vi "CNR find scaling parameters.vi"(10 "parameters":dbl[](array[numeric]), 11 "old parameter scale factors":dbl[](array[numeric])) -> (3 "parameter scale factors":dbl[](array[numeric]))   [LabVIEW 2017, in "NI_Gmath.lvlib"]
uses:
  <vilib>/gmath/NI_Gmath.lvlib
panel:
  in  "scale params?":bool=TRUE
  out "x*y":dbl[](array[numeric])
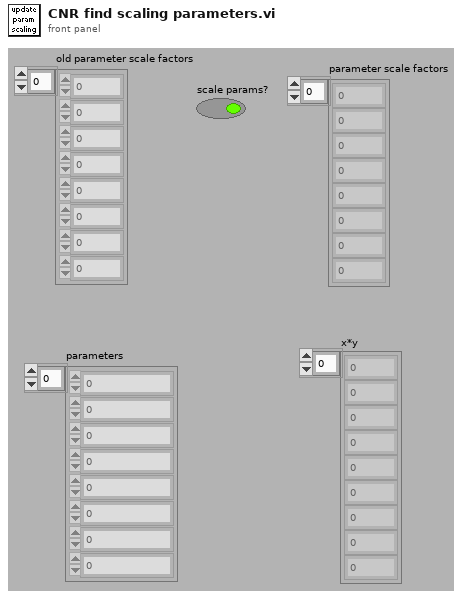
[diagram p1: front panel]
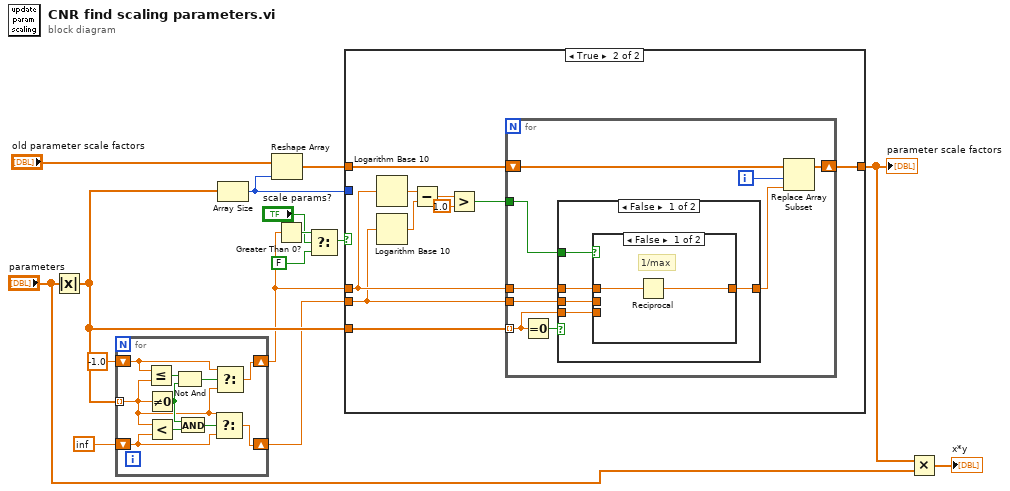
[diagram p0: block diagram]
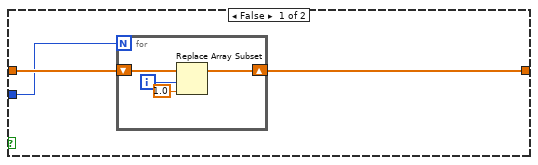
[diagram p2: hidden frame]
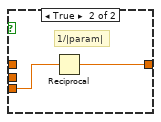
[diagram p3: hidden frame]
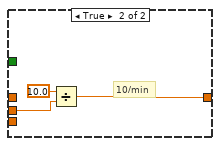
[diagram p4: hidden frame]
diagram:
  n1 = Absolute Value(x="parameters") -> (abs(x)=w12:dbl[])
  n2 = for {
    tunnel: w12 -> [w16] mode=indexing
    shift-right: [w19] -> w8
    shift-left: -1.0 ("y") -> [w17]
    shift-right: [w18] -> w9
    shift-left: inf -> [w20]
    n3 = Less Or Equal?(x=w17, y=w16) -> (x <= y?=w25:bool)
    n4 = Not Equal To 0?(x=w16) -> (x != 0?=w24:bool)
    n5 = Less?(x=w16, y=w20) -> (x < y?=w23:bool)
    n6 = Not And(1:w24, 2:w25) -> (0:w22:bool)
    n7 = And(x=w24, y=w23) -> (x .and. y?=w21:bool)
    n8 = Select(t=w16, s=w21, f=w20) -> (s? t:f=w18:dbl)
    n9 = Select(t=w17, s=w22, f=w16) -> (s? t:f=w19:dbl)
  }
  n10 = Array Size(array=w12) -> (size(s)=w15:i32)
  n11 = Reshape Array("old parameter scale factors", w15) -> (w13:dbl[])
  n12 = Greater Than 0?(x=w8) -> (x > 0?=w2:bool)
  n13 = Select(t=w2, s="scale params?", f=FALSE) -> (s? t:f=w3:bool)
  n14 = case shown="True" w3 {
    tunnel: w15 -> [w27 _]
    tunnel: w8 -> [_ w36]
    tunnel: w9 -> [_ w35]
    tunnel: w12 -> [_ w42]
    tunnel: w13 -> [w28 w34]
    tunnel: [w26 w33] -> w7
    frame False {
      n15 = for {
        N: w27 -> [_]
        shift-right: [w31] -> w26
        shift-left: w28 -> [w32]
        i -> [w30]
        n16 = Replace Array Subset(array=w32, new element=1.0 ("element"), index=w30) -> (w31:dbl[])
      }
    }
    frame True {
      n17 = Logarithm Base 10(1:w36) -> (0:w41:dbl)
      n18 = Logarithm Base 10(1:w35) -> (0:w40:dbl)
      n19 = Subtract(x=w41, y=w40) -> (x-y=w39:dbl)
      n20 = Greater?(x=w39, y=1.0) -> (0:w37:bool)
      n21 = for {
        tunnel: w42 -> [w46] mode=indexing
        tunnel: w37 -> [w43]
        tunnel: w36 -> [w47]
        tunnel: w35 -> [w48]
        shift-right: [w50] -> w33
        shift-left: w34 -> [w51]
        i -> [w44]
        n22 = Equal To 0?(x=w46) -> (x = 0?=w49:bool)
        n23 = case shown="False" w49 {
          tunnel: w48 -> [w54 w62]
          tunnel: w47 -> [w55 _]
          tunnel: w46 -> [w53 _]
          tunnel: [w52 w61] -> w45
          tunnel: w43 -> [w56 _]
          frame False {
            n24 = case shown="False" w56 {
              tunnel: w55 -> [w58 _]
              tunnel: w54 -> [_ _]
              tunnel: w53 -> [_ w60]
              tunnel: [w57 w59] -> w52
              frame False {
                # "1/max"
                n25 = Reciprocal(x=w58) -> (1/x=w57:dbl)
              }
              frame True {
                # "1/|param|"
                n26 = Reciprocal(x=w60) -> (1/x=w59:dbl)
              }
            }
          }
          frame True {
            # "10/min"
            n27 = Divide(x=10.0, y=w62) -> (x/y=w61:dbl)
          }
        }
        n28 = Replace Array Subset(array=w51, new element=w45, index=w44) -> (w50:dbl[])
      }
    }
  }
  "parameter scale factors" <- w7
  n29 = Multiply(x=w7, y="parameters") -> (x*y=→"x*y":dbl[])
